vi "DAQ - Get wForms for File Save.vi"(0 "reference in":refnum<class "GSwFormDSP.lvclass">, 5 "error in (no error)":errorcluster, 6 "Reset Buffer OFFSET":bool) -> (11 "t0":timestamp, 13 "wForms for FILE":waveform(dbl)[](array[waveform]), 14 "reference out":refnum<class "GSwFormDSP.lvclass">, 19 "error out":errorcluster)   [LabVIEW 2022 SP3, in "GSwFormDSP.lvclass"]
uses:
  GSwFormDSP.lvclass
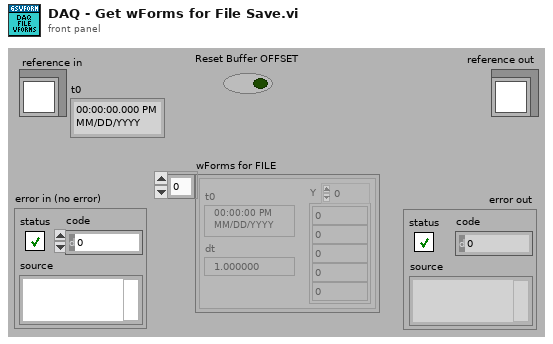
[diagram p1: front panel]
types:
  T1 = typedef "GSwFormDSP.lvclass/ObjectAttributes.ctl" = cluster{"Wform Ref":refnum<data-value>, "Nb Signals":i32, "Spectral Function Parameters":T2, "FFT":waveform(cdb)[], "Nb FFT":i32, "Nb Averages":i32[], "Reference Indexes":i32[], "Response Indexes":i32[], "Coherence":waveform(dbl)[], "TDF Parameters":T4, "DAQ":cluster{"Duration (sec)":dbl, "Buffer Size (Samples)":i32, "Offset (Samples)":i32}, "Filter Impulse Response (TDF)":waveform(dbl), "Sound Playback":T5}
  T2 = typedef "GSwFormDSP.lvclass/Spectral Parameters.ctl" = cluster{"Frequency resolution (Hz)":dbl, "Overlap":dbl, "Window":T3}
  T3 = typedef "NI_AALPro.lvlib/windowTd.ctl" = u32
  T4 = typedef "GSwFormDSP.lvclass/TDF Parameters.ctl" = cluster{"Filter":enum32{"Lowpass", "Highpass", "Bandpass", "Bandstop"}, "Type:":enum16{"Butterworth", "Chebyshev", "Inv Chebyshev", "Elliptic", "Bessel"}, "LP cutoff freq":dbl, "HP cutoff freq":dbl, "Order":i32, "passband ripple (dB)":dbl, "stopband attenuation (dB)":dbl, "Phaseless Filter":bool, "Include Fade IN and OUT":bool}
  T5 = typedef "GSwFormDSP.lvclass/Sound Playback.ctl" = cluster{"Timer start (ms)":u32, "task ID":T6, "Cursor Init Location (s)":dbl, "SC Volume":dbl}
  T6 = typedef "Sound Output Task ID.ctl" = u32
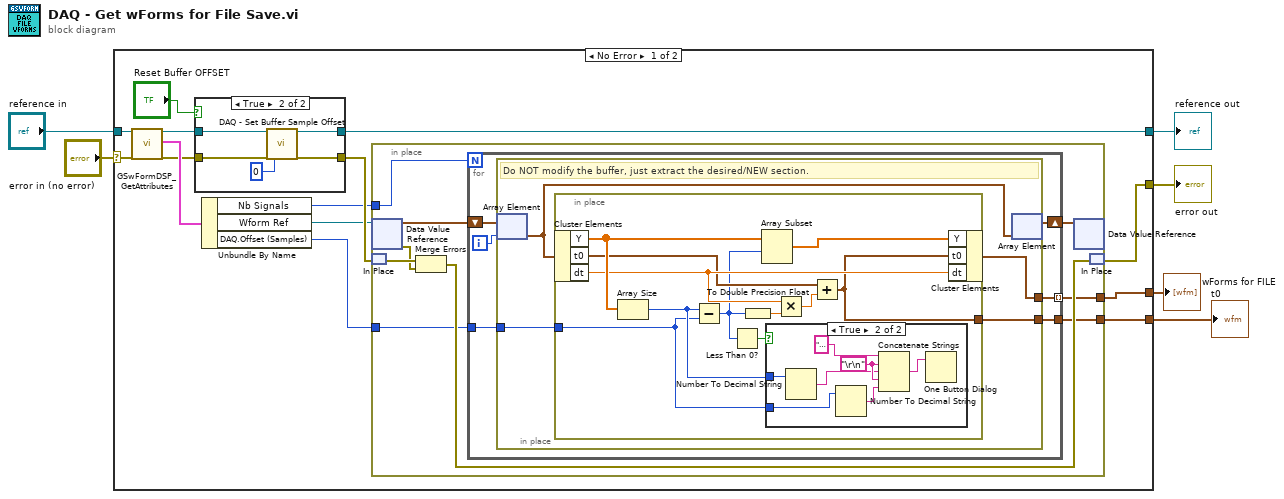
[diagram p0: block diagram]
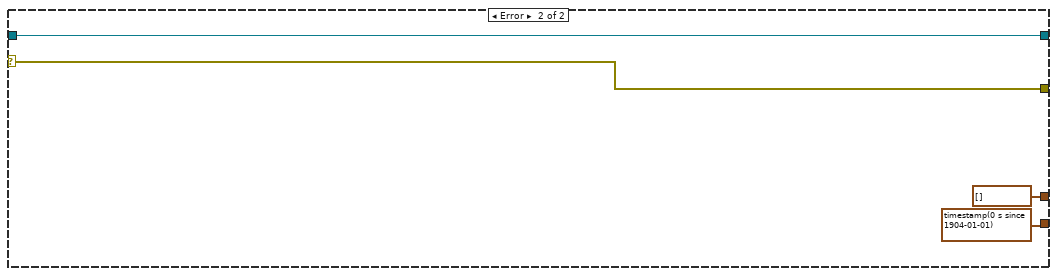
[diagram p4: hidden frame]
diagram:
  n1 = case shown="No Error" "error in (no error)" {
    selector: "error in (no error)" -> [w20 w68]
    tunnel: [w10 w68] -> w5
    tunnel: [w12 w67] -> w3
    tunnel: "reference in" -> [w19 w67]
    tunnel: [w11 timestamp(0 s since 1904-01-01)] -> w2
    tunnel: [w9 waveform(dbl)[] []] -> w1
    frame No Error {
      n2 = call "GSwFormDSP_GetAttributes.vi"("reference in"=w19, "error in (no error)"=w20) -> ("reference out"=w17:refnum<class "GSwFormDSP.lvclass">, "attributes"=w18:T1, "error out"=w15:errorcluster)  [unwired: 14 in, 1 out]
      n3 = case shown="True" "Reset Buffer OFFSET" {
        tunnel: w17 -> [w22 w27]
        tunnel: [w21 w25] -> w16
        tunnel: w15 -> [w21 w24]
        tunnel: [w22 w23] -> w12
        frame False {
        }
        frame True {
          n4 = call "DAQ - Set Buffer Sample Offset.vi"("reference in"=w27, "error in (no error)"=w24, "DAQ.Offset (Samples)"=0) -> ("reference out"=w23:refnum<class "GSwFormDSP.lvclass">, "error out"=w25:errorcluster)  [unwired: 15 in]
        }
      }
      n5 = Unbundle By Name(w18) -> ("Nb Signals"=w8:i32, "Wform Ref"=w13:refnum<data-value>, "DAQ.Offset (Samples)"=w14:i32)
      n6 = in-place {
        in-place-border: w14 -> [w32]
        in-place-border: [w30] -> w9
        in-place-border: [w29] -> w11
        in-place-border: w8 -> [w28]
        n7 = in-place-dvr #1(w13) -> (w31:waveform(dbl)[], w34:errorcluster)
        n8 = in-place-match #2(w16) -> (w35:errorcluster)
        n9 = Merge Errors(w35, w34) -> (w36:errorcluster)
        n10 = for {
          N: w28 -> [_]
          shift-right: [w41] -> w33
          shift-left: w31 -> [w42]
          tunnel: w32 -> [w38]
          tunnel: [w40] -> w30 mode=indexing
          tunnel: [w37] -> w29
          i -> [w39]
          n11 = in-place {
            in-place-border: [w45] -> w40
            in-place-border: w38 -> [w46]
            in-place-border: [w43] -> w37
            # "Do NOT modify the buffer, just extract the desired/NEW section."
            n12 = in-place-array #3(w42, w39) -> (w44:waveform(dbl))
            n13 = in-place {
              in-place-border: w46 -> [w47]
              in-place-border: [w49] -> w43
              n14 = in-place-cluster #4(w44) -> ("Y"=w57:dbl[], "t0"=w52:timestamp, "dt"=w54:dbl)
              n15 = Array Size(array=w57) -> (size(s)=w48:i32)
              n16 = Subtract(x=w48, y=w47) -> (x-y=w51:i32)
              n17 = Less Than 0?(x=w51) -> (x < 0?=w50:bool)
              n18 = To Double Precision Float(number=w51) -> (double precision float=w55:dbl)
              n19 = Array Subset(array=w57, index=w51) -> (w56:dbl[])  [unwired: 1 in]
              n20 = case shown="True" w50 {
                tunnel: w48 -> [_ w61]
                tunnel: w47 -> [_ w58]
                frame False {
                }
                frame True {
                  w62 = "\r\n"
                  n21 = Number To Decimal String(number=w61) -> (decimal integer string=w60:string)  [unwired: 1 in]
                  n22 = Number To Decimal String(number=w58) -> (decimal integer string=w59:string)  [unwired: 1 in]
                  n23 = Concatenate Strings("Something is wrong with the \"Get wForms for File Save vi\".  the current sample index is greater than the buffer size???", w62, w60, w62, w59) -> (w63:string)
                  n24 = One Button Dialog(message=w63) -> ()  [unwired: 1 in, 1 out]
                }
              }
              n25 = Multiply(x=w54, y=w55) -> (x*y=w53:dbl)
              n26 = Add(x=w52, y=w53) -> (x+y=w49:timestamp)
              n27 = in-place-cluster #4("Y"=w56, "t0"=w49, "dt"=w54) -> (w45:waveform(dbl))
            }
            n28 = in-place-array #3(w44) -> (w41:waveform(dbl)[])  [unwired: 1 out]
          }
        }
        n29 = in-place-dvr #1(w33) -> ()  [unwired: 2 out]
        n30 = in-place-match #2(w36) -> (w10:errorcluster)
      }
    }
    frame Error {
    }
  }
  "error out" <- w5
  "reference out" <- w3
  "t0" <- w2
  "wForms for FILE" <- w1
